vi "LED Config (3 colors built in)vi.vi"(8 "refnum name":string, 9 "Channel C":bool, 10 "Channel B":bool, 11 "Channel A":bool) -> ()   [LabVIEW 2019]
uses:
  <vilib>/Rock Robotics/WPI/ThirdParty/Phoenix-LabVIEW/CANifier/CTRE_CANifier_LEDChannel.ctl
  Documents/GitHub/MARS-2020/mOS_XIII/MoS_XIII/Globals/LED_Globals.vi
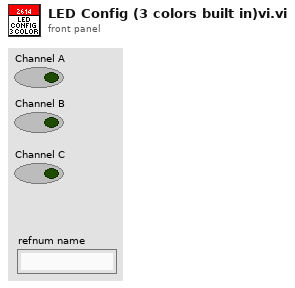
[diagram p1: front panel]
types:
  T1 = typedef "CTRE_CANifier_LEDChannel.ctl" = enum32{"LEDChannelA", "LEDChannelB", "LEDChannelC"}
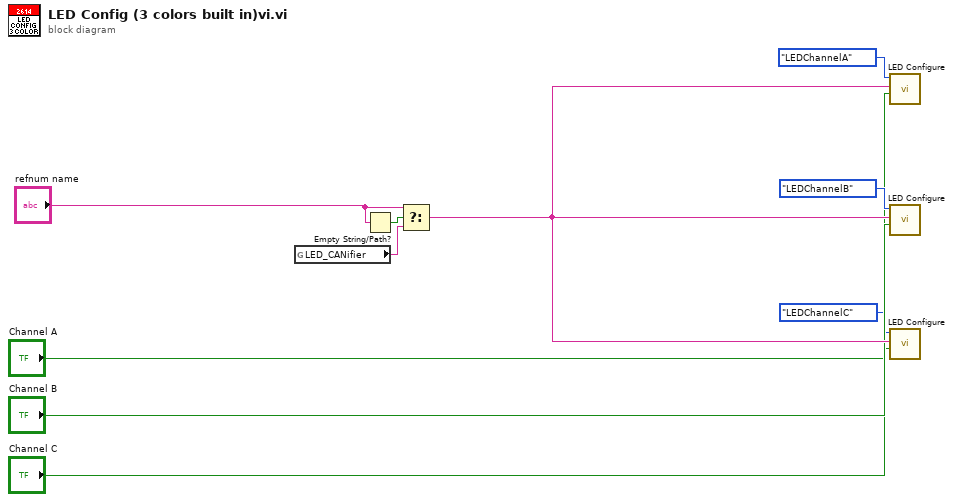
[diagram p0: block diagram]
diagram:
  n1 = global read "LED_Globals.vi" "LED_CANifier"() -> (w9:string)
  n2 = Empty String/Path?(string/path="refnum name") -> (empty?=w7:bool)
  n3 = Select(t="refnum name", s=w7, f=w9) -> (s? t:f=w8:string)
  n4 = call "LED Configure.vi"("LED On"="Channel A", "refnum name"=w8, "LEDChannel"=CTRE_CANifier_LEDChannel."LEDChannelA") -> ()  [unwired: 9 in]
  n5 = call "LED Configure.vi"("LED On"="Channel B", "refnum name"=w8, "LEDChannel"=CTRE_CANifier_LEDChannel."LEDChannelB") -> ()  [unwired: 9 in]
  n6 = call "LED Configure.vi"("LED On"="Channel C", "refnum name"=w8, "LEDChannel"=CTRE_CANifier_LEDChannel."LEDChannelC") -> ()  [unwired: 9 in]
